vi "Build_Scatter_Data.vi"(8 "Rising Index":i32[](array[numeric]), 11 "PMT (AI 0)":u8[](graph)) -> (2 "data":cluster{"x":dbl, "y":dbl}[](array[cluster]) {"y" format="%.2f"; "x" format="%.2f"})   [LabVIEW 2012]
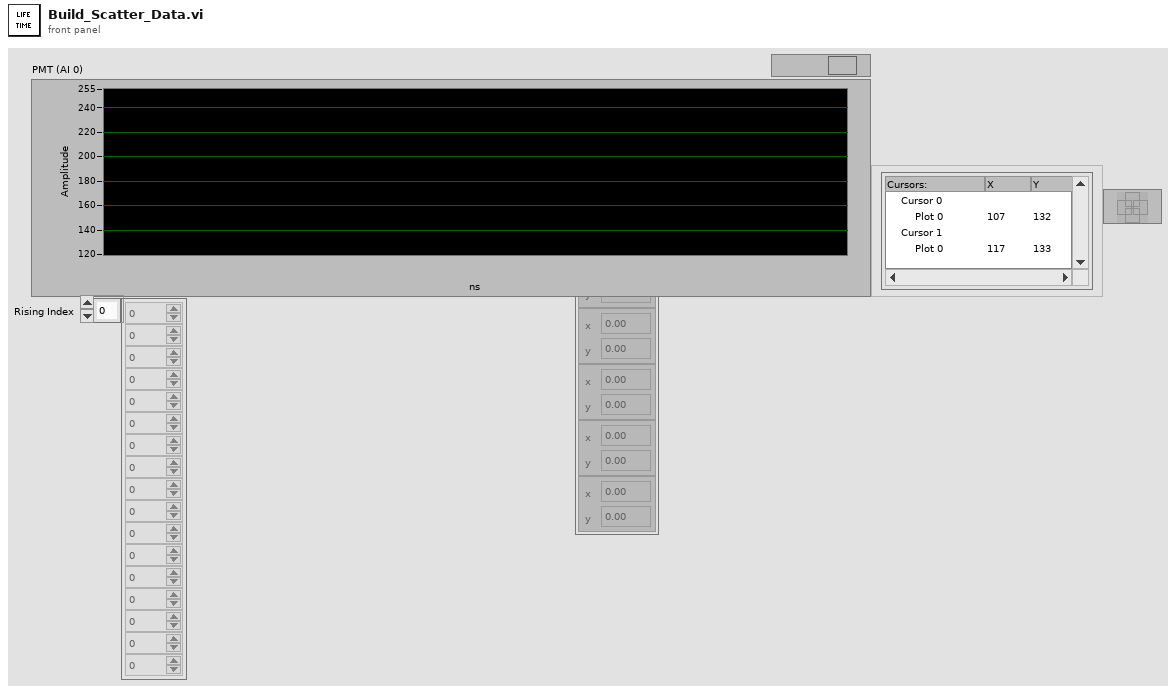
[diagram p1: front panel]
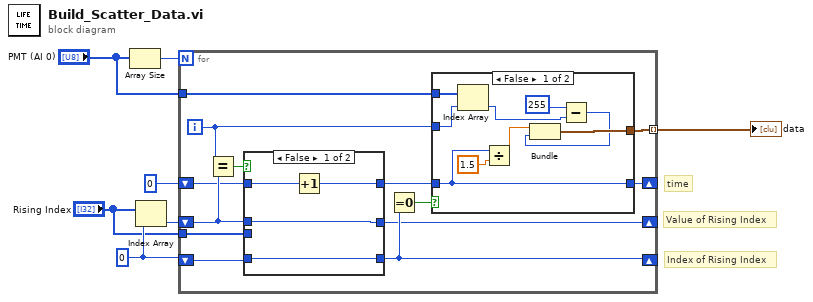
[diagram p0: block diagram]
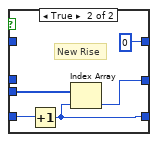
[diagram p2: hidden frame]
diagram:
  w6 = 0
  # "time"
  # "Value of Rising Index"
  # "Index of Rising Index"
  n1 = Array Size(array="PMT (AI 0)") -> (size(s)=w7:i32)
  n2 = Index Array(array="Rising Index", index=w6) -> (element=w5:i32)
  n3 = for {
    N: w7 -> [_]
    tunnel: [w20] -> w1 mode=indexing
    shift-right: [w16] -> _
    shift-left: w6 -> [w17]
    shift-right: [w14] -> _
    shift-left: w5 -> [w12]
    tunnel: "Rising Index" -> [w15]
    shift-right: [w9] -> _
    shift-left: 0 -> [w11]
    tunnel: "PMT (AI 0)" -> [w8]
    i -> [w13]
    n4 = Equal?(x=w13, y=w12) -> (x = y?=w18:bool)
    n5 = case shown="False" w18 {
      tunnel: w17 -> [w24 w29]
      tunnel: [w24 w27] -> w16
      tunnel: w15 -> [_ w28]
      tunnel: [w23 w26] -> w14
      tunnel: w12 -> [w23 _]
      tunnel: w11 -> [w22 _]
      tunnel: [w21 0] -> w10
      frame False {
        n6 = Increment(x=w22) -> (x+1=w21:i32)
      }
      frame True {
        # "New Rise"
        n7 = Increment(x=w29) -> (x+1=w27:i32)
        n8 = Index Array(array=w28, index=w27) -> (element=w26:i32)
      }
    }
    n9 = Equal To 0?(x=w16) -> (x = 0?=w19:bool)
    n10 = case shown="False" w19 {
      tunnel: w13 -> [w34 _]
      tunnel: [w38 _] -> w20
      tunnel: w10 -> [w37 w39]
      tunnel: [w37 w39] -> w9
      tunnel: w8 -> [w35 _]
      frame False {
        n11 = Index Array(array=w35, index=w34) -> (element=w31:u8)
        n12 = Divide(x=w37, y=1.5) -> (x/y=w33:dbl)
        n13 = Subtract(x=255, y=w31) -> (x-y=w30:i32)
        n14 = Bundle(w33, w30) -> (w38:cluster{dbl, i32})  [unwired: 1 in]
      }
      frame True {
      }
    }
  }
  "data" <- w1
